vi "TemplateBehavior.vi"(3 "SupressIn":dbl, 7 "Inhibit":bool, 8 "HowAmI? Clean":cluster{"T":dbl, "Battery":dbl, "Temp":dbl}, 9 "WhatAroundMe? Clean":cluster{"T":dbl, "Range":dbl, "Bearing":dbl}[](array[cluster]), 10 "WhereAmI? Clean":T1, 11 "Velocity":dbl) -> (0 "SupressOut":dbl, 2 "ActCommand":dbl[](array[numeric]), 4 "InhibitOut":bool)   [LabVIEW 2010]
doc: "This subVI acta as a template for Midbrain behaviors. Its inputs are the outputs of teh three SENSE processes, the overall velocity requested of the robot, a suppression value from another co-brahvior and an inhibit signal to turn the behavior off. The outputs are a 90 element steering array and a suppression value to diminish the output of co-behaviors.\n\nIt is designed to work with a 90 element behavior arbiter."
panel:
  # "This VI is a template for creating a robot subbehavior at the Midbrain level"
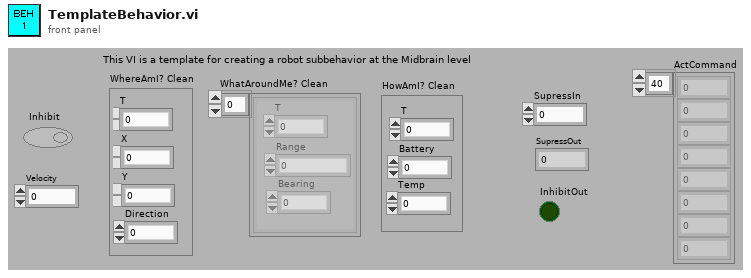
[diagram p1: front panel]
types:
  T1 = cluster{"T":dbl, "X":dbl, "Y":dbl, "Direction":dbl}
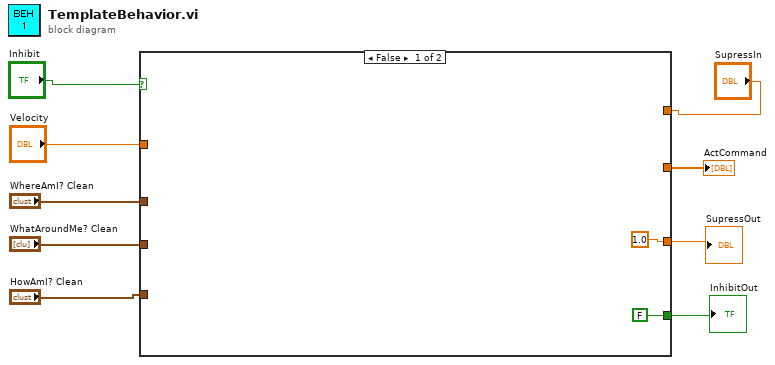
[diagram p0: block diagram]
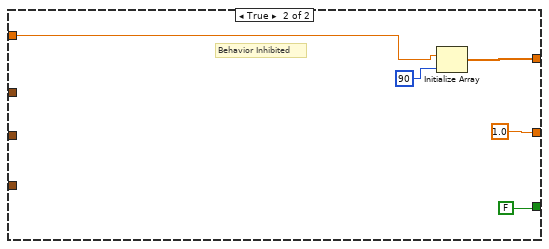
[diagram p2: hidden frame]
diagram:
  n1 = case shown="False" "Inhibit" {
    tunnel: "Velocity" -> [_ w12]
    tunnel: "WhatAroundMe? Clean" -> [_ _]
    tunnel: "WhereAmI? Clean" -> [_ _]
    tunnel: "HowAmI? Clean" -> [_ _]
    tunnel: "SupressIn" -> [_ _]
    tunnel: [_ w14] -> w2
    tunnel: [1.0 ("SupressOut") 1.0 ("SupressOut")] -> w3
    tunnel: [FALSE ("InhibitOut") FALSE ("InhibitOut")] -> w1
    frame False {
    }
    frame True {
      # "Behavior Inhibited"
      n2 = Initialize Array "Initialize Array"(w12, 90 ("dimension size")) -> (w14:dbl[])
    }
  }
  "ActCommand" <- w2
  "SupressOut" <- w3
  "InhibitOut" <- w1
